vi "01 - Single.vi"() -> ()   [LabVIEW 2019]
uses:
  Grassfire/Direction--enum.ctl
  Grassfire/Solution--cluster.ctl
  Grassfire/Solution--picture ring.ctl
  Grassfire/Selection--2D array.ctl
  Grassfire/Selection--picture ring.ctl
  Grassfire/Grassfire.lvclass
panel:
  in  "Selection Grid":T1=[[{"Grid Value"=0}, {"Grid Value"=0}, {"Grid Value"=0}, {"Grid Value"=0}, {"Grid Value"=0}, {"Grid Value"=0}, {"Grid Value"=0}, {"Grid Value"=0}], [{"Grid Value"=0}, {"Grid Value"=2}, {"Grid Value"=0}, {"Grid Value"=1}, {"Grid Value"=0}, {"Grid Value"=0}, {"Grid Value"=0}, {"Grid Value"=0}], [{"Grid Value"=0}, {"Grid Value"=0}, {"Grid Value"=0}, {"Grid Value"=0}, {"Grid Value"=0}, {"Grid Value"=0}, {"Grid Value"=0}, {"Grid Value"=0}], [{"Grid Value"=0}, {"Grid Value"=0}, {"Grid Value"=1}, {"Grid Value"=0}, {"Grid Value"=0}, {"Grid Value"=0}, {"Grid Value"=0}, {"Grid Value"=0}], [{"Grid Value"=0}, {"Grid Value"=1}, {"Grid Value"=0}, {"Grid Value"=0}, {"Grid Value"=1}, {"Grid Value"=0}, {"Grid Value"=0}, {"Grid Value"=0}], [{"Grid Value"=0}, {"Grid Value"=0}, {"Grid Value"=0}, {"Grid Value"=1}, {"Grid Value"=1}, {"Grid Value"=1}, {"Grid Value"=1}, {"Grid Value"=0}], [{"Grid Value"=0}, {"Grid Value"=0}, {"Grid Value"=0}, {"Grid Value"=0}, {"Grid Value"=0}, {"Grid Value"=0}, {"Grid Value"=0}, {"Grid Value"=0}], [{"Grid Value"=0}, {"Grid Value"=0}, {"Grid Value"=0}, {"Grid Value"=0}, {"Grid Value"=0}, {"Grid Value"=3}, {"Grid Value"=0}, {"Grid Value"=0}], [{"Grid Value"=0}, {"Grid Value"=0}, {"Grid Value"=0}, {"Grid Value"=0}, {"Grid Value"=0}, {"Grid Value"=0}, {"Grid Value"=0}, {"Grid Value"=0}]]
  in  "Heading":T3=enum."Down"
  out "Valid":bool
  out "Directions":T3[](array[typedef])
  out "Solution Grid":T4[][](array[typedef])
  # "1. Edit Selection Grid\n2. Run VI"
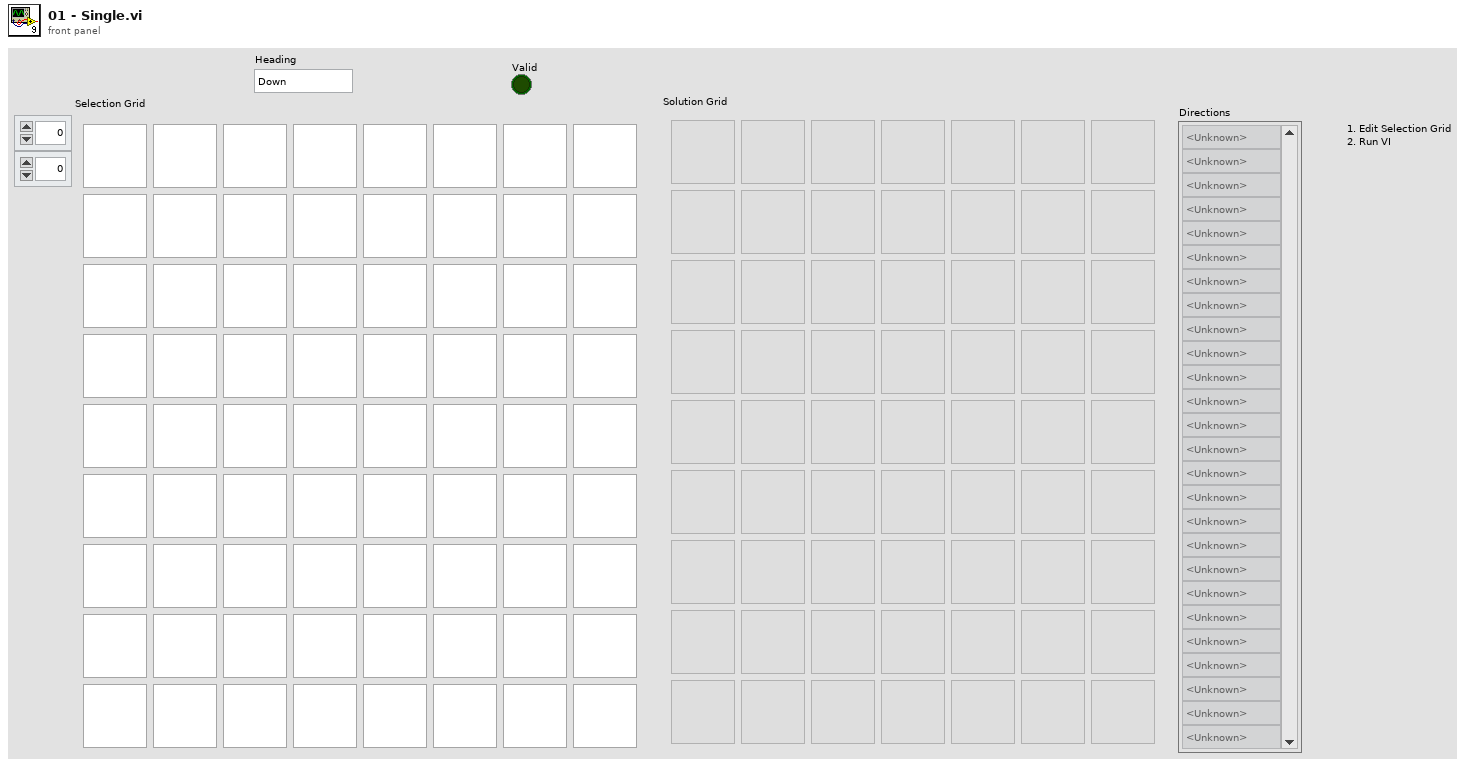
[diagram p1: front panel]
types:
  T1 = typedef "Grassfire.lvclass/Selection--2D array.ctl" = cluster{"Grid Value":T2}[][]
  T2 = typedef "Grassfire.lvclass/Selection--picture ring.ctl" = i64
  T3 = typedef "Grassfire.lvclass/Direction--enum.ctl" = enum16{"<Unknown>", "Right", "Down", "Left", "Up"}
  T4 = typedef "Grassfire.lvclass/Solution--cluster.ctl" = cluster{"Node Type":T5, "Distance":string}
  T5 = typedef "Grassfire.lvclass/Solution--picture ring.ctl" = i64
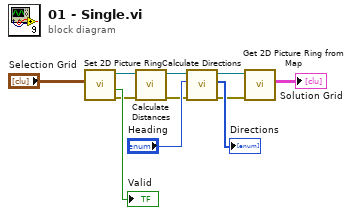
[diagram p0: block diagram]
diagram:
  n1 = call "Set 2D Picture Ring.vi"("Selection Grid"="Selection Grid") -> ("error out"=w3:errorcluster, "Valid"=→"Valid":bool, "Grassfire out"=w7:refnum<class "Grassfire.lvclass">)  [unwired: 8 in]
  n2 = call-dynamic "Calculate Distances.vi"("error in (no error)"=w3, "Grassfire in"=w7) -> ("error out"=w2:errorcluster, "Grassfire out"=w10:refnum<class "Grassfire.lvclass">)  [unwired: 8 in]
  n3 = call-dynamic "Calculate Directions.vi"("error in (no error)"=w2, "Heading"="Heading", "Grassfire in"=w10) -> ("error out"=w1:errorcluster, "Directions"=→"Directions":T3[], "Grassfire out"=w11:refnum<class "Grassfire.lvclass">)  [unwired: 6 in]
  n4 = call-dynamic "Get 2D Picture Ring from Map.vi"("error in (no error)"=w1, "Grassfire in"=w11) -> ("Array"=→"Solution Grid":T4[][])  [unwired: 7 in, 2 out]
